vi "Exercise2.vi"() -> ()   [LabVIEW 2019]
uses:
  <vilib>/Utility/error.llb/DialogType.ctl
  <vilib>/DAQmx/write.llb/DAQmx Write (Analog DBL 1Chan 1Samp).vi
  <vilib>/DAQmx/create/channels.llb/DAQmx Create Channel (AO-Voltage-Basic).vi
  <vilib>/DAQmx/miscellaneous.llb/DAQmx Fill In Error Info.vi
panel:
  in  "Motor 2":dbl(slide) caption="Motor 2 (Lx - left)" scale=-10.0..10.0
  in  "Maximum voltage 2":dbl
  in  "Minimum Voltage 2":dbl
  in  "DAQmx Physical Channel 2":tag="Dev1/ai0"
  in  "stop 2":bool
  in  "Maximum voltage":dbl
  in  "Minimum Voltage":dbl
  in  "DAQmx Physical Channel":tag="Dev1/ai0"
  in  "Motor 1":dbl(slide) caption="Motor 1 (Rx - right)" scale=-10.0..10.0
  in  "stop":bool
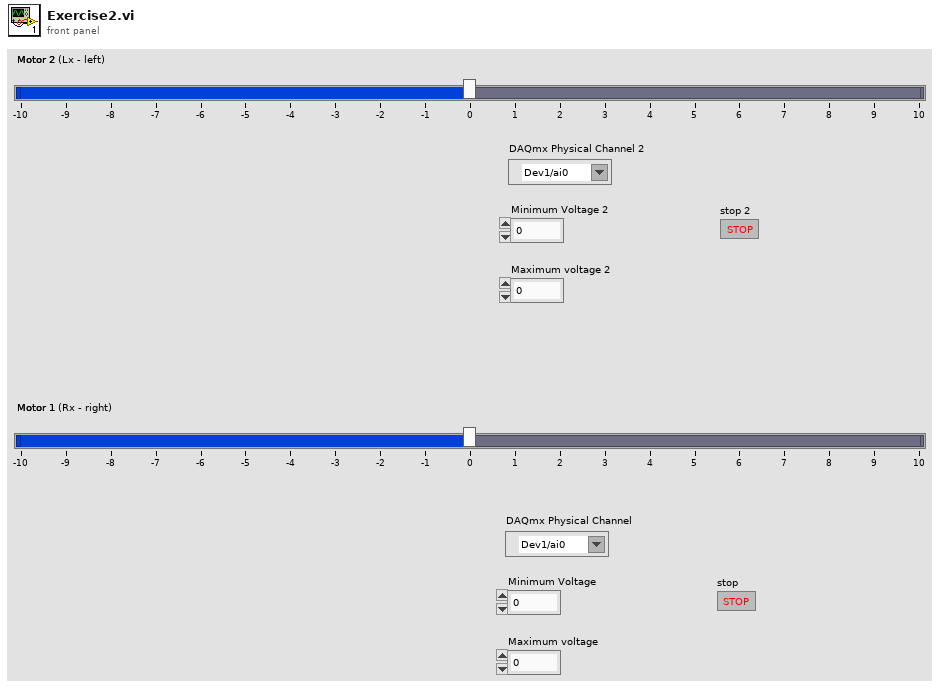
[diagram p1: front panel]
types:
  T1 = typedef "DialogType.ctl" = u16
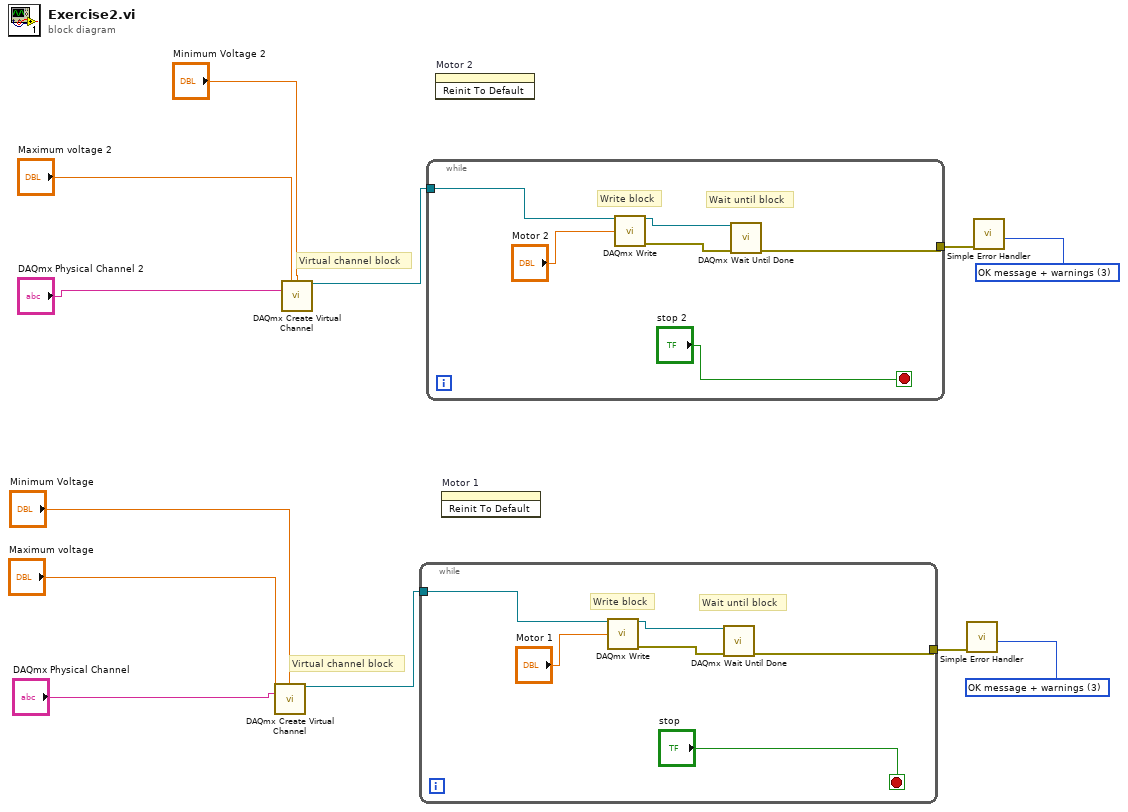
[diagram p0: block diagram]
diagram:
  w6 = T1 3 items=["no dialog", "OK message", "continue or stop message", "OK message + warnings", "continue/stop + warnings"] ("type of dialog (OK msg:1)")
  w12 = T1 3 items=["no dialog", "OK message", "continue or stop message", "OK message + warnings", "continue/stop + warnings"] ("type of dialog (OK msg:1)")
  # "Virtual channel block"
  # "Virtual channel block"
  n1 = call-poly <vilib>:"DAQmx Create Virtual Channel.vi"("maximum value"="Maximum voltage", "minimum value"="Minimum Voltage", "physical channels"="DAQmx Physical Channel") -> ("task out"=w8:refnum<k21>)  [unwired: 11 in, 1 out]
  n2 = call-poly <vilib>:"DAQmx Create Virtual Channel.vi"("maximum value"="Maximum voltage 2", "minimum value"="Minimum Voltage 2", "physical channels"="DAQmx Physical Channel 2") -> ("task out"=w5:refnum<k21>)  [unwired: 11 in, 1 out]
  n3 = while {
    tunnel: w8 -> [w17]
    tunnel: [w14] -> w7
    stop <- "stop" stop-if-true
    # "Wait until block"
    # "Write block"
    n4 = call-poly <vilib>:"DAQmx Write.vi"("task/channels in"=w17, "data"="Motor 1") -> ("task out"=w16:refnum<k21>, "error out"=w15:errorcluster)  [unwired: 11 in, 1 out]
    n5 = call <vilib>:"DAQmx Wait Until Done.vi"("task/channels in"=w16, "error in"=w15) -> ("error out"=w14:errorcluster)  [unwired: 12 in, 1 out]
  }
  n6 = while {
    tunnel: w5 -> [w24]
    tunnel: [w21] -> w4
    stop <- "stop 2" stop-if-true
    # "Wait until block"
    # "Write block"
    n7 = call-poly <vilib>:"DAQmx Write.vi"("task/channels in"=w24, "data"="Motor 2") -> ("task out"=w23:refnum<k21>, "error out"=w22:errorcluster)  [unwired: 11 in, 1 out]
    n8 = call <vilib>:"DAQmx Wait Until Done.vi"("task/channels in"=w23, "error in"=w22) -> ("error out"=w21:errorcluster)  [unwired: 12 in, 1 out]
  }
  n9 = invoke on="Motor 2" class="Slide (strict)" method="Reinit To Default"() -> ()  [unwired: 3 in, 3 out]
  n10 = invoke on="Motor 1" class="Slide (strict)" method="Reinit To Default"() -> ()  [unwired: 3 in, 3 out]
  n11 = call <vilib>:"Simple Error Handler.vi"("type of dialog (OK msg:1)"=w12, "error in (no error)"=w7) -> ()  [unwired: 3 in, 5 out]
  n12 = call <vilib>:"Simple Error Handler.vi"("type of dialog (OK msg:1)"=w6, "error in (no error)"=w4) -> ()  [unwired: 3 in, 5 out]
